vi "close connection.vi"(8 "error in (no error)":errorcluster, 11 "tcp server in":refnum<class "tcp connection.lvclass">) -> (0 "error out":errorcluster, 3 "tcp server out":refnum<class "tcp connection.lvclass">)   [LabVIEW 2014, in "tcp connection.lvclass"]
doc: "This vi will execute normally even if there is an incoming error."
uses:
  tcp connection.lvclass
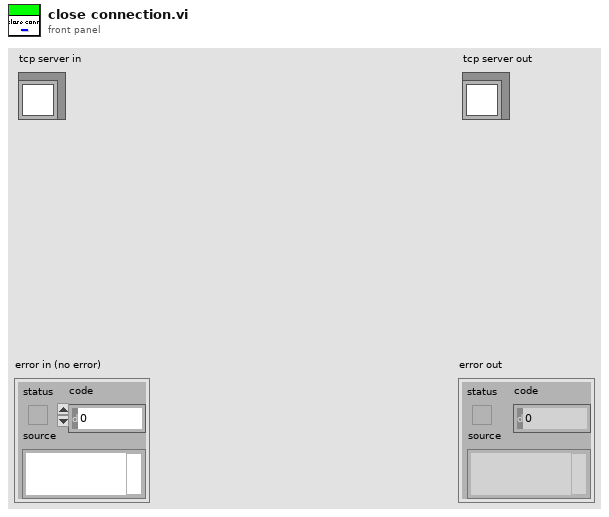
[diagram p1: front panel]
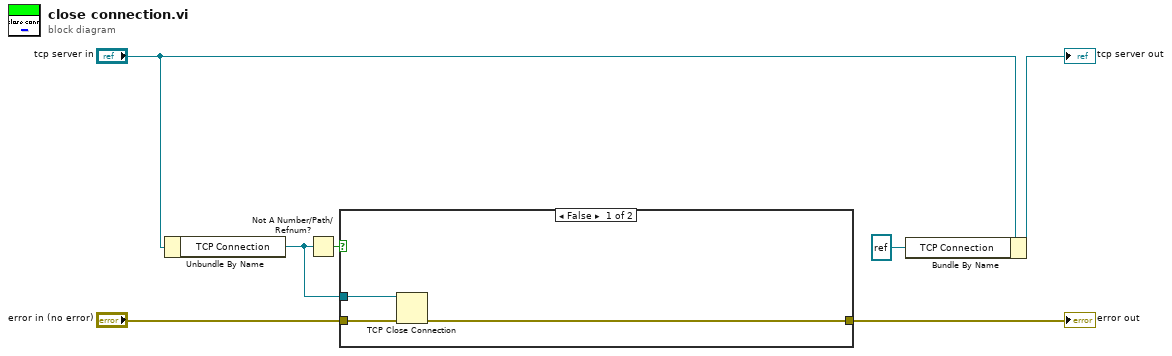
[diagram p0: block diagram]
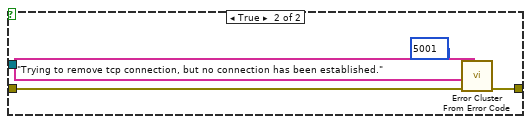
[diagram p2: hidden frame]
diagram:
  n1 = Unbundle By Name("tcp server in") -> ("TCP Connection"=w2:refnum<k5>)
  n2 = Not A Number/Path/Refnum?(number/path/refnum=w2) -> (NaN/Path/Refnum?=w3:bool)
  n3 = case shown="False" w3 {
    tunnel: w2 -> [w10 _]
    tunnel: "error in (no error)" -> [w9 w12]
    tunnel: [w8 w11] -> w6
    frame False {
      n4 = TCP Close Connection(connection ID=w10, error in (no error)=w9) -> (error out=w8:errorcluster)  [unwired: 1 in, 1 out]
    }
    frame True {
      n5 = call <vilib>:"Error Cluster From Error Code.vi"("error in (no error)"=w12, "error message (\"\")"="Trying to remove tcp connection, but no connection has been established." ("error message (\"\")"), "error code (0)"=5001) -> ("error out"=w11:errorcluster)  [unwired: 6 in]
    }
  }
  "error out" <- w6
  n6 = Bundle By Name(cluster="tcp server in", "TCP Connection"=refnum<k5> refnum ("TCP Network Connection in")) -> (→"tcp server out":refnum<class "tcp connection.lvclass">)
